vi "Globals.vi"() -> ()   [LabVIEW 2023]
panel:
  in  "Digitals Transfer Done":bool
  in  "Analogues Transfer Done":bool
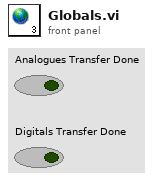
[diagram p1: front panel]
diagram:
